vi "displayFitsImage16.vi"(8 "error in (no error)":errorcluster, 11 "filename":string="C:\\Users\\tiba\\Desktop\\fits\\image8.fits") -> (0 "error out":errorcluster, 1 "Error message":string, 2 "FITS image":picture, 3 "filename dup":string, 5 "OK":bool)   [LabVIEW 2019]
uses:
  <vilib>/picture/picture.llb/Draw 8-Bit Pixmap.vi
  F:/INO340/OSL/FITSdemo/fits/lib/testfits.dll
panel:
  out "size (in bytes)":i64
  # "1164 *  880"
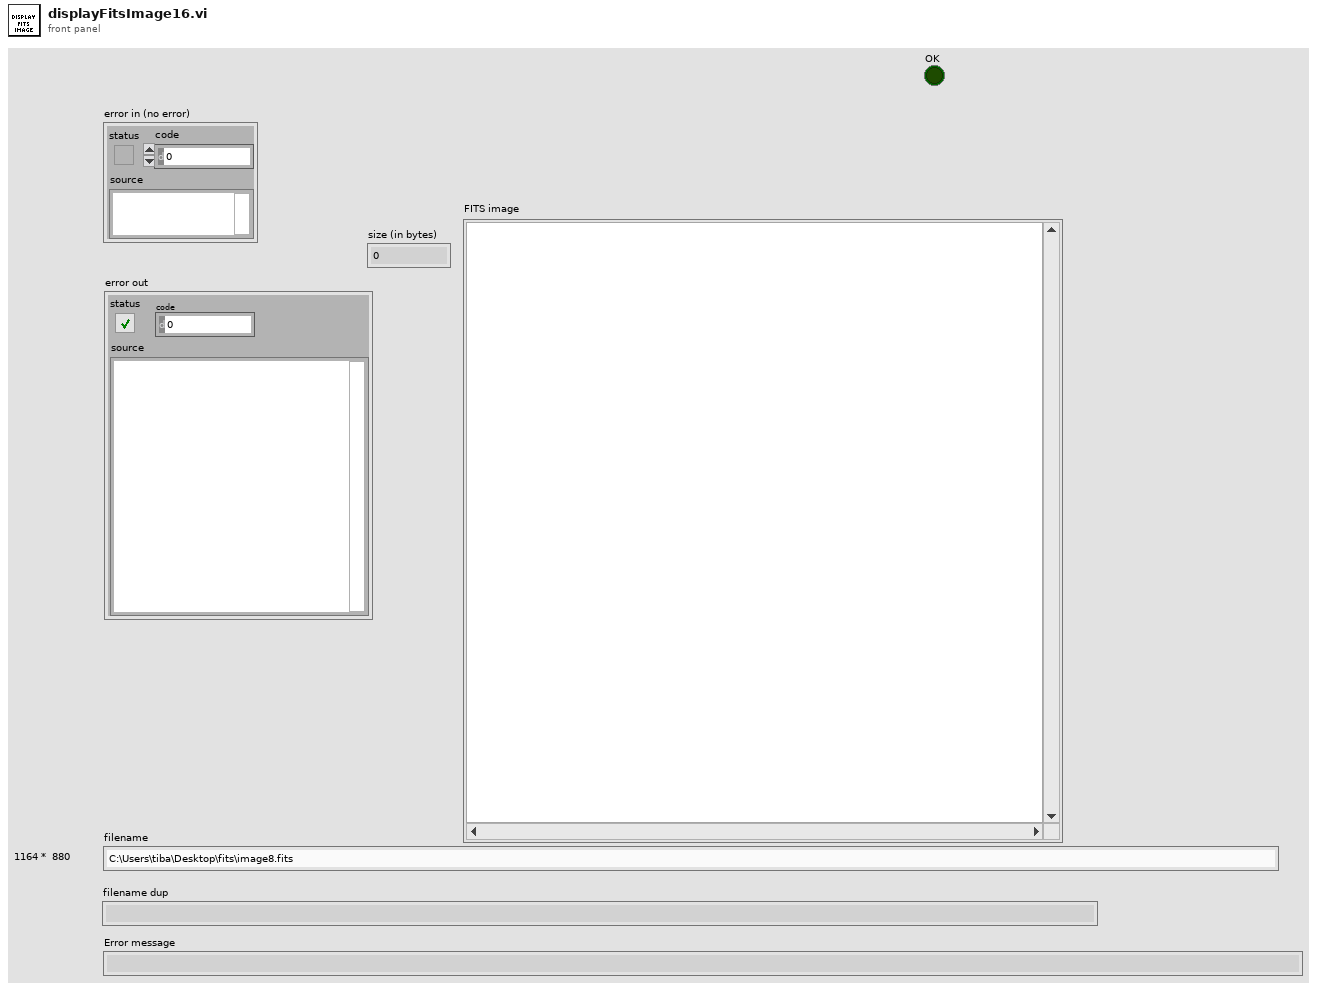
[diagram p1: front panel]
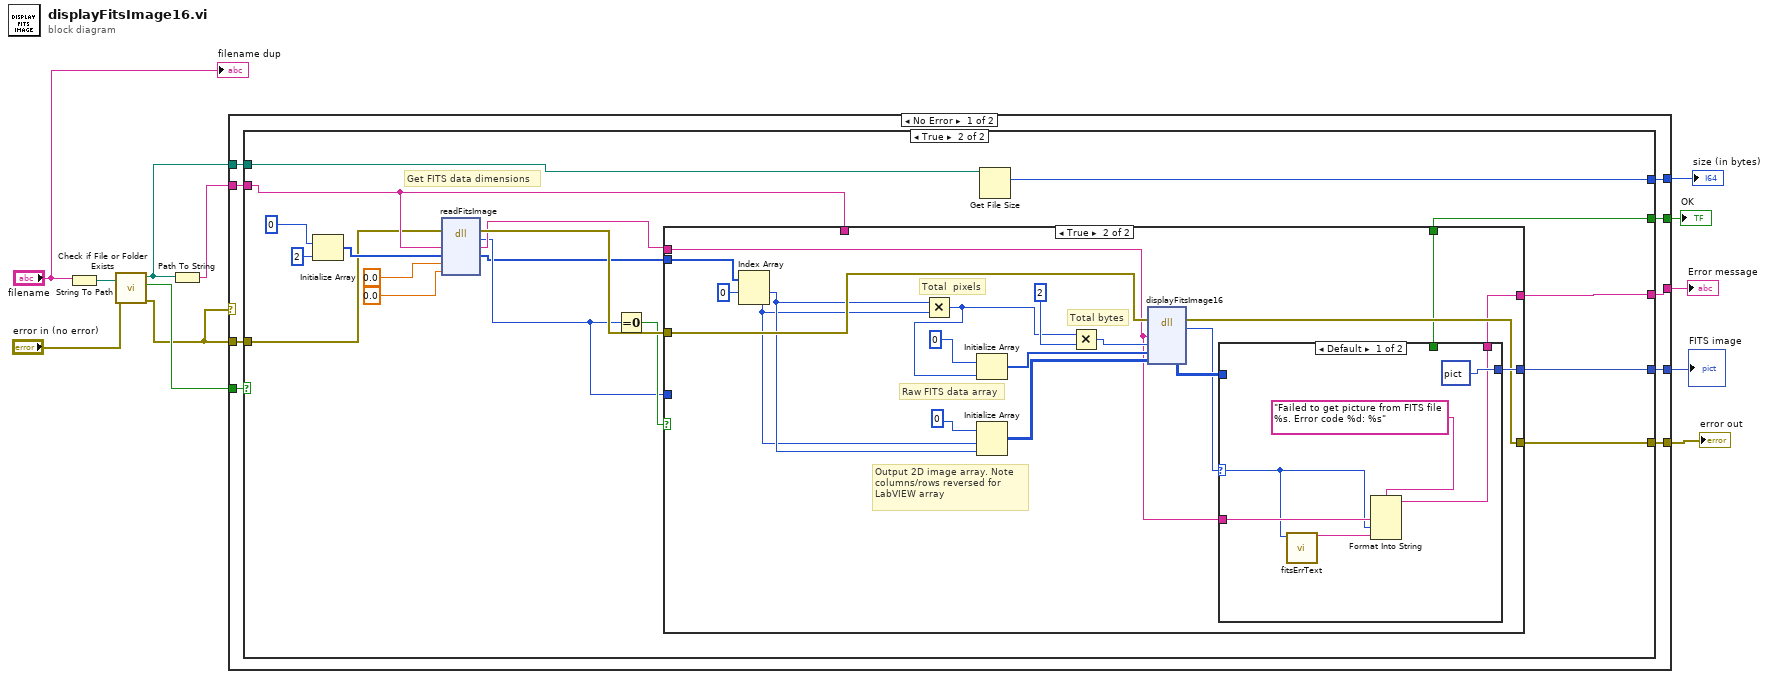
[diagram p0: block diagram]
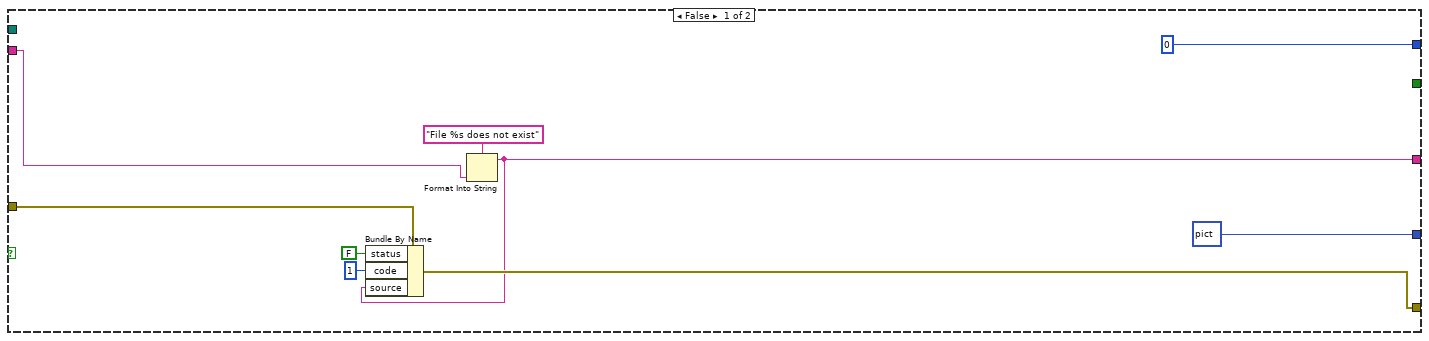
[diagram p2: hidden frame]
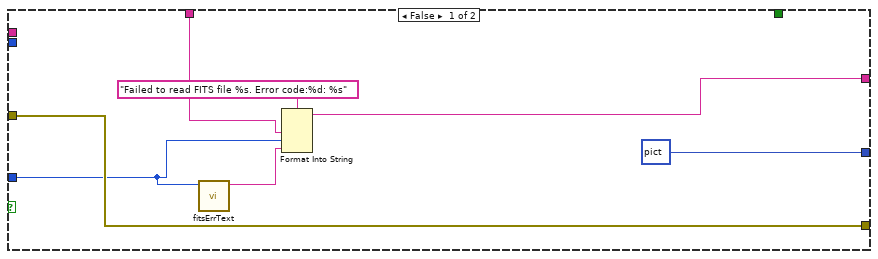
[diagram p3: hidden frame]
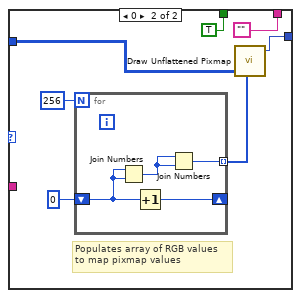
[diagram p4: hidden frame]
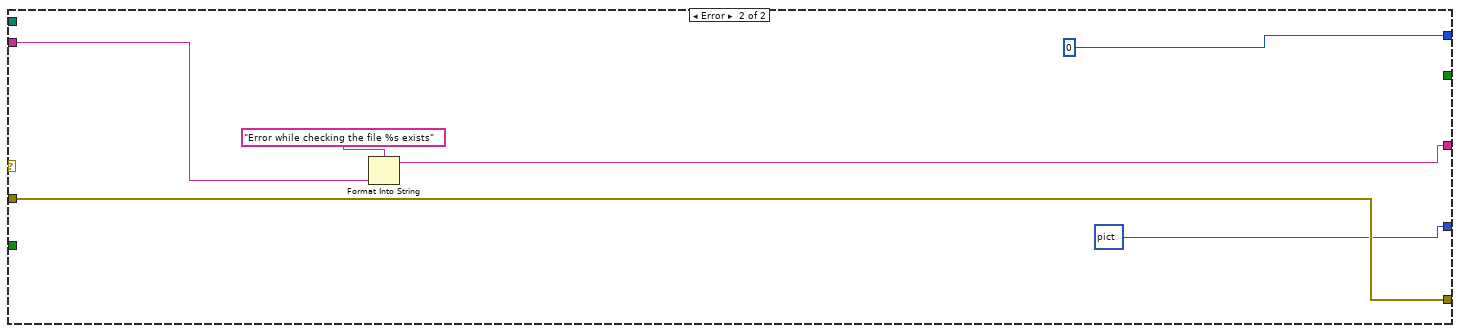
[diagram p5: hidden frame]
diagram:
  n1 = String To Path(string="filename") -> (path=w11:path)
  n2 = call <vilib>:"Check if File or Folder Exists.vi"("error in (no error)"="error in (no error)", "path"=w11) -> ("error out"=w2:errorcluster, "file or folder exists?"=w9:bool, "dup path"=w8:path)  [unwired: 7 in]
  n3 = Path To String(path=w8) -> (string=w10:string)
  n4 = case shown="No Error" w2 {
    tunnel: w10 -> [w21 w95]
    tunnel: w9 -> [w20 _]
    tunnel: w8 -> [w19 _]
    tunnel: w2 -> [w18 w97]
    tunnel: [w17 i64 0 ("size (in bytes)")] -> w6
    tunnel: [w16 w94] -> w5
    tunnel: [w15 picture data[5B] ("new picture")] -> w4
    tunnel: [w14 w97] -> w3
    tunnel: [w13 _] -> w1
    frame No Error {
      n5 = case shown="True" w20 {
        tunnel: w21 -> [w26 w40]
        tunnel: w19 -> [_ w39]
        tunnel: w18 -> [w27 w34]
        tunnel: [i64 0 ("size (in bytes)") w38] -> w17
        tunnel: [w22 w37] -> w16
        tunnel: [picture data[5B] ("new picture") w36] -> w15
        tunnel: [w23 w35] -> w14
        tunnel: [_ w33] -> w13
        frame False {
          n6 = Format Into String(format string="File %s does not exist", w26) -> (resulting string=w22:string)  [unwired: 2 in, 1 out]
          n7 = Bundle By Name(cluster=w27, "status"=FALSE, "code"=1, "source"=w22) -> (w23:errorcluster)
        }
        frame True {
          # "Get FITS data dimensions"
          n8 = Initialize Array(0 ("element"), 2 ("dimension size")) -> (w46:i32[])
          n9 = dll-call lib="F:/INO340/OSL/FITSdemo/fits/lib/testfits.dll" fn="readFitsImage"(error in=w34, "filename"=w40, "npix"=w46, "dmin"=sgl 0.0, "dmax"=sgl 0.0) -> (error out=w43:errorcluster, "return type"=w32:i32, "filename"=w41:string, "npix"=w31:i32[])  [unwired: 4 in, 1 out]
          n10 = Equal To 0?(x=w32) -> (x = 0?=w42:bool)
          n11 = case shown="True" w42 {
            tunnel: w43 -> [w51 w66]
            tunnel: w41 -> [_ w61]
            tunnel: w40 -> [w54 _]
            tunnel: [w53 w60] -> w37
            tunnel: [picture data[5B] ("new picture") w65] -> w36
            tunnel: [w51 w64] -> w35
            tunnel: [_ w62] -> w33
            tunnel: w32 -> [w49 _]
            tunnel: w31 -> [_ w59]
            frame False {
              n12 = call "fitsErrText.vi"("status"=w49) -> ("message"=w50:string)  [unwired: 10 in]
              n13 = Format Into String(format string="Failed to read FITS file %s. Error code:%d: %s", w54, w49, w50) -> (resulting string=w53:string)  [unwired: 2 in, 1 out]
            }
            frame True {
              # "Raw FITS data array"
              # "Output 2D image array. Note\ncolumns/rows reversed for\nLabVIEW array"
              # "Total bytes"
              # "Total  pixels"
              n14 = Index Array(array=w59, index #1=0 ("index")) -> (element #1=w57:i32, element #2=w56:i32)  [unwired: 1 in]
              n15 = Multiply(x=w57, y=w56) -> (x*y=w68:i32)
              n16 = Initialize Array(0 ("element"), w68) -> (w73:i32[])
              n17 = Initialize Array(u8 0 ("element"), w56, w57) -> (w69:u8[][])
              n18 = Multiply(x=w68, y=2 ("Bytes per pixel")) -> (x*y=w72:i32)
              n19 = dll-call lib="F:/INO340/OSL/FITSdemo/fits/lib/testfits.dll" fn="displayFitsImage16"(error in=w66, "filename"=w61, "isize"=w72, "img"=w73, "outdat"=w69) -> (error out=w64:errorcluster, "return type"=w63:i32, "outdat"=w67:u8[][])  [unwired: 5 in, 1 out]
              n20 = case shown="Default" w63 {
                selector: w63 -> [w76 _]
                tunnel: w67 -> [_ w84]
                tunnel: [picture data[5B] ("new picture") w83] -> w65
                tunnel: [_ TRUE] -> w62
                tunnel: w61 -> [w78 _]
                tunnel: [w77 ""] -> w60
                frame Default {
                  n21 = call "fitsErrText.vi"("status"=w76) -> ("message"=w75:string)  [unwired: 10 in]
                  n22 = Format Into String(format string="Failed to get picture from FITS file %s. Error code %d: %s", w78, w76, w75) -> (resulting string=w77:string)  [unwired: 2 in, 1 out]
                }
                frame 0 {
                  # "Populates array of RGB values\nto map pixmap values"
                  n23 = for {
                    N: 256 -> [_]
                    tunnel: [w91] -> w85 mode=indexing
                    shift-right: [w90] -> _
                    shift-left: u8 0 -> [w88]
                    n24 = Join Numbers(hi=w88, lo=w88) -> ((hi.lo)=w89:u16)
                    n25 = Increment(x=w88) -> (x+1=w90:u8)
                    n26 = Join Numbers(hi=w89, lo=w89) -> ((hi.lo)=w91:u32)
                  }
                  n27 = call-poly <vilib>:"Draw Unflattened Pixmap.vi"("data"=w84, "color table"=w85) -> ("new picture"=w83:picture)  [unwired: 7 in]
                }
              }
            }
          }
          n28 = Get File Size(file=w39) -> (size (in bytes)=w38:i64)  [unwired: 1 in, 2 out]
        }
      }
    }
    frame Error {
      n29 = Format Into String(format string="Error while checking the file %s exists", w95) -> (resulting string=w94:string)  [unwired: 2 in, 1 out]
    }
  }
  "size (in bytes)" <- w6
  "Error message" <- w5
  "FITS image" <- w4
  "error out" <- w3
  "OK" <- w1
  "filename dup" <- "filename"
